vi "Read Version.vi"(8 "error in (no error)":errorcluster, 11 "Version Data in":refnum<class "Version Data.lvclass">) -> (0 "error out":errorcluster, 2 "Build Specification Version":T1, 3 "Version Data out":refnum<class "Version Data.lvclass">)   [LabVIEW 2019, in "ProjectBuilder.lvlib" / "Version Data.lvclass"]
doc: "Read version data."
uses:
  Version Data.lvclass
  <vilib>/AppBuilder/AB_API_Simple/Build Specification Version.ctl
  <vilib>/AppBuilder/AB_API_Simple/NI_App_Builder_API.lvlib
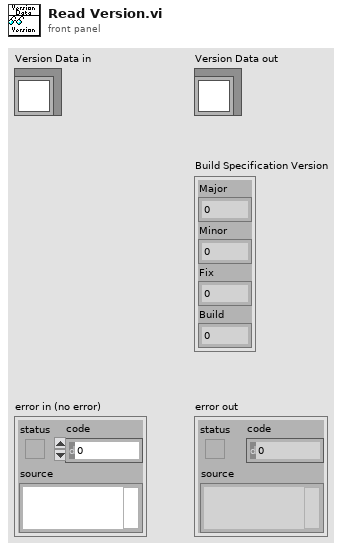
[diagram p1: front panel]
types:
  T1 = typedef "NI_App_Builder_API.lvlib/Build Specification Version.ctl" = cluster{"Major":u16, "Minor":u16, "Fix":u16, "Build":u16}
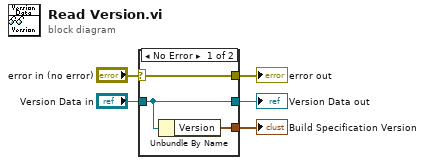
[diagram p0: block diagram]
diagram:
  n1 = case shown="No Error" "error in (no error)" {
    selector: "error in (no error)" -> [w8 w9]
    tunnel: [w8 w9] -> w4
    tunnel: [w7 w10] -> w2
    tunnel: "Version Data in" -> [w7 w10]
    tunnel: [w6 _] -> w1
    frame No Error {
      n2 = Unbundle By Name(w7) -> ("Version"=w6:T1)
    }
    frame Error {
    }
  }
  "error out" <- w4
  "Version Data out" <- w2
  "Build Specification Version" <- w1
